vi "getTaskChannel.vi"(8 "error in (no error)":errorcluster, 11 "TaskMock in":refnum<class "TaskMock.lvclass">) -> (0 "error out":errorcluster, 2 "taskChannel":refnum<class "ITaskChannel.lvclass">, 3 "TaskMock out":refnum<class "TaskMock.lvclass">)   [LabVIEW 2023, in "TaskMock.lvclass"]
doc: "Returns the Task Channel type used by the task."
uses:
  source/ITaskChannel/ITaskChannel.lvclass
  TaskMock.lvclass
  TaskMock.lvclass/TaskMock.ctl
  source/BoolNotifierTaskChannel/BoolNotifierTaskChannel.lvclass
  C:/projects/TLC_Daemon/source/BoolNotifierTaskChannel/BoolNotifierTaskChannel.lvclass
  C:/projects/TLC_Daemon/source/ITaskChannel/ITaskChannel.lvclass
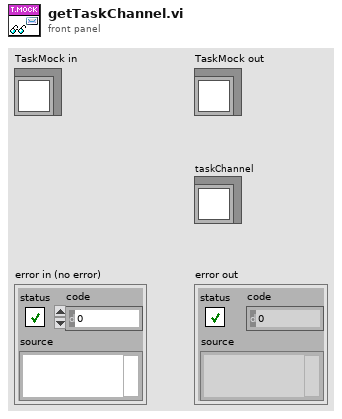
[diagram p1: front panel]
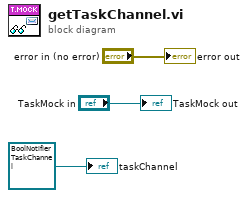
[diagram p0: block diagram]
diagram:
  "error out" <- "error in (no error)"
  "TaskMock out" <- "TaskMock in"
  "taskChannel" <- refnum<class "BoolNotifierTaskChannel.lvclass"> refnum ("TLC_Daemon.lvlib:BoolNotifierTaskChannel.lvclass")
